vi "Run-Time Menu - Create entries for module--helper.vi"(7 "Menu in":refnum<k9>, 8 "error in":errorcluster, 10 "Module Descriptor":string, 11 "Module DQMH Path":path) -> (0 "error out":errorcluster)   [LabVIEW 2022 SP3, in "UI Manager.lvlib"]
doc: "____\nHAMPEL SOFTWARE ENGINEERING v2.6.0 (2023-12-19 10:54)"
uses:
  UI Manager.lvlib
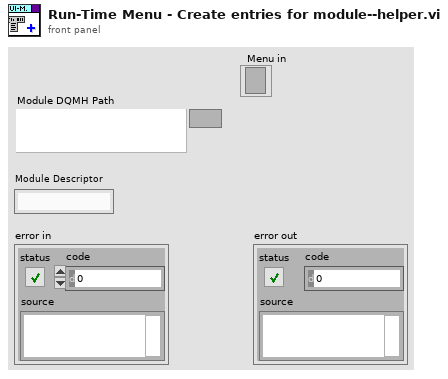
[diagram p1: front panel]
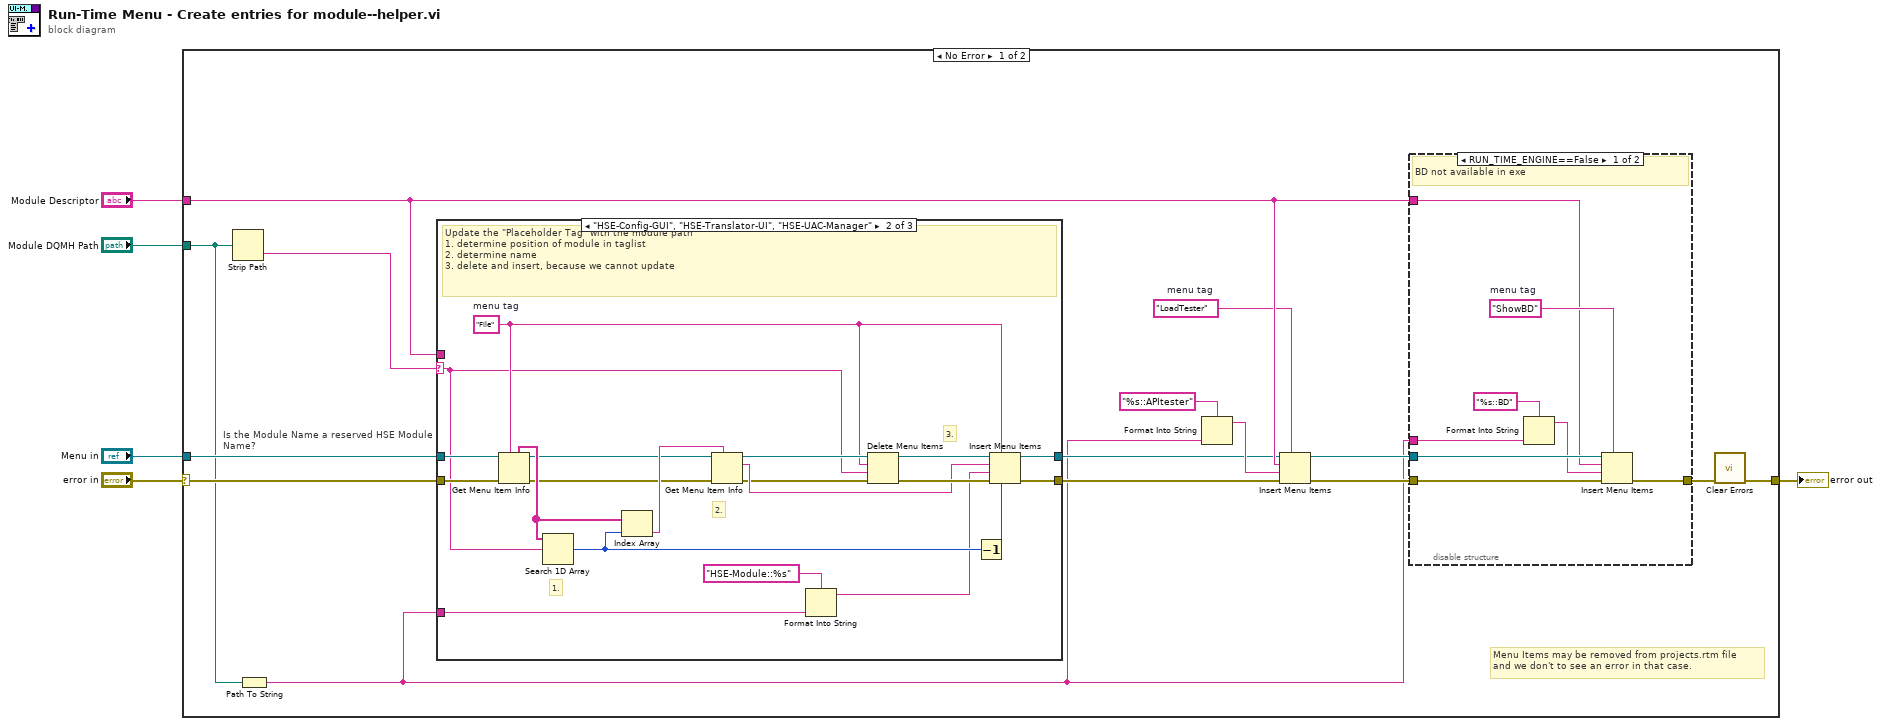
[diagram p0: block diagram]
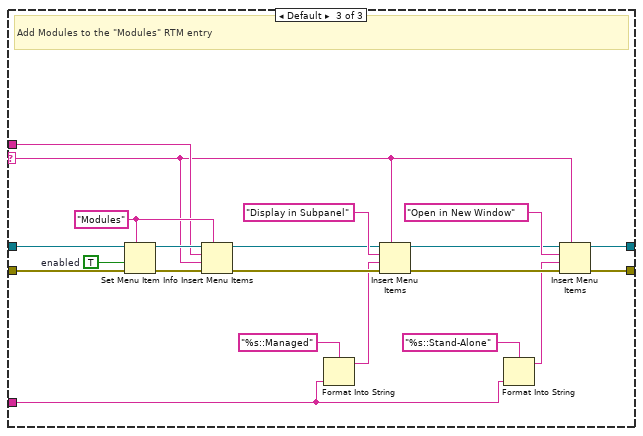
[diagram p3: hidden frame]
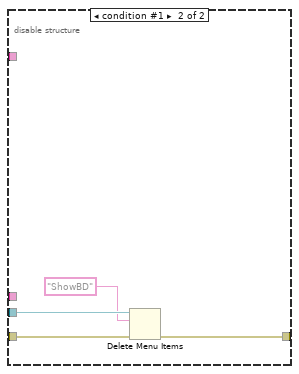
[diagram p4: hidden frame]
diagram:
  n1 = case shown="No Error" "error in" {
    selector: "error in" -> [w11 w76]
    tunnel: [w8 w76] -> w5
    tunnel: "Module DQMH Path" -> [w10 _]
    tunnel: "Menu in" -> [w20 _]
    tunnel: "Module Descriptor" -> [w19 _]
    frame No Error {
      w16 = "LoadTester"  # menu tag
      # "Menu Items may be removed from projects.rtm file\nand we don't to see an error in that case."
      n2 = Strip Path(path=w10) -> (name=w6:string)  [unwired: 1 out]
      n3 = Path To String(path=w10) -> (string=w9:string)
      n4 = case "Is the Module Name a reserved HSE Module Name?" shown="\"HSE-Config-GUI\", \"HSE-Translator-UI\", \"HSE-UAC-Manager\"" w6 {
        selector: w6 -> [_ w23 w43]
        tunnel: w20 -> [w21 w37 w61]
        tunnel: w11 -> [w22 w38 w59]
        tunnel: [w21 w39 w47] -> w15
        tunnel: [w22 w40 w46] -> w14
        tunnel: w19 -> [_ _ w45]
        tunnel: w9 -> [_ w24 w44]
        frame "Event Manager", "Navigation", "UI Manager" {
          # "Do not add Framework modules to the \"Modules\" RTM entry"
        }
        frame "HSE-Config-GUI", "HSE-Translator-UI", "HSE-UAC-Manager" {
          w27 = "File"  # menu tag
          # "3."
          # "2."
          # "1."
          # "Update the \"Placeholder Tag\" with the module path\n1. determine position of module in taglist\n2. determine name\n3. delete and insert, because we cannot update"
          n5 = Get Menu Item Info(7:w27, 8:w38, 11:w37) -> (0:w29:errorcluster, 3:w31:refnum<k9>, 5:w35:string[])  [unwired: 4 out]
          n6 = Search 1D Array(1D array=w35, element=w23) -> (index of element=w34:i32)  [unwired: 1 in]
          n7 = Index Array(array=w35, index=w34) -> (element=w33:string)
          n8 = Get Menu Item Info(7:w33, 8:w29, 11:w31) -> (0:w28:errorcluster, 2:w32:string, 3:w30:refnum<k9>)  [unwired: 4 out]
          n9 = Format Into String(format string="HSE-Module::%s", w24) -> (resulting string=w25:string)  [unwired: 2 in, 1 out]
          n10 = Delete Menu Items(6:w28, 7:w23, 8:w27, 9:w30) -> (0:w41:errorcluster, 3:w42:refnum<k9>)
          n11 = Decrement(x=w34) -> (x-1=w36:i32)
          n12 = Insert Menu Items(4:w36, 5:w27, 6:w41, 7:w25, 8:w32, 9:w42) -> (0:w40:errorcluster, 3:w39:refnum<k9>)  [unwired: 1 out]
        }
        frame Default {
          w62 = TRUE  # enabled
          w63 = "Modules" ("menu tag")
          # "Add Modules to the \"Modules\" RTM entry"
          n13 = Set Menu Item Info(7:w63, 8:w59, 9:w62, 11:w61) -> (0:w58:errorcluster, 3:w60:refnum<k9>)  [unwired: 3 in]
          n14 = Insert Menu Items(5:w63, 6:w58, 7:w43, 8:w45, 9:w60) -> (0:w55:errorcluster, 3:w54:refnum<k9>)  [unwired: 1 in, 1 out]
          n15 = Format Into String(format string="%s::Managed", w44) -> (resulting string=w48:string)  [unwired: 2 in, 1 out]
          n16 = Insert Menu Items(5:w43, 6:w55, 7:w48, 8:"Display in Subpanel" ("string"), 9:w54) -> (0:w52:errorcluster, 3:w53:refnum<k9>)  [unwired: 1 in, 1 out]
          n17 = Format Into String(format string="%s::Stand-Alone", w44) -> (resulting string=w49:string)  [unwired: 2 in, 1 out]
          n18 = Insert Menu Items(5:w43, 6:w52, 7:w49, 8:"Open in New Window" ("string"), 9:w53) -> (0:w46:errorcluster, 3:w47:refnum<k9>)  [unwired: 1 in, 1 out]
        }
      }
      n19 = Format Into String(format string="%s::APItester", w9) -> (resulting string=w18:string)  [unwired: 2 in, 1 out]
      n20 = Insert Menu Items(5:w16, 6:w14, 7:w18, 8:w19, 9:w15) -> (0:w12:errorcluster, 3:w13:refnum<k9>)  [unwired: 1 in, 1 out]
      n21 = disable-structure shown="RUN_TIME_ENGINE==False" {
        disable-tunnel: w13 -> [w70 w75]
        disable-tunnel: w12 -> [w69 w74]
        disable-tunnel: [w71 w73] -> w7
        disable-tunnel: w9 -> [w65 _]
        disable-tunnel: w19 -> [w64 _]
        frame condition #0 (active) {
          w68 = "ShowBD"  # menu tag
          # "BD not available in exe"
          n22 = Format Into String(format string="%s::BD", w65) -> (resulting string=w66:string)  [unwired: 2 in, 1 out]
          n23 = Insert Menu Items(5:w68, 6:w69, 7:w66, 8:w64, 9:w70) -> (0:w71:errorcluster)  [unwired: 1 in, 2 out]
        }
        frame condition #1 {
          n24 = Delete Menu Items(6:w74, 8:"ShowBD" ("menu tag"), 9:w75) -> (0:w73:errorcluster)  [unwired: 1 in, 1 out]
        }
      }
      n25 = call <vilib>:"Clear Errors.vi"("error in (no error)"=w7) -> ("error out"=w8:errorcluster)  [unwired: 5 in, 1 out]
    }
    frame Error {
    }
  }
  "error out" <- w5
